vi "Write Stick Deadband.vi"(8 "error in (no error)":errorcluster, 10 "Stick Deadband":dbl, 11 "Joystick in":refnum<class "Joystick.lvclass">) -> (0 "error out":errorcluster, 3 "Joystick out":refnum<class "Joystick.lvclass">)   [LabVIEW 2014, in "Joystick.lvlib" / "Joystick.lvclass"]
uses:
  Joystick.lvclass
  Joystick.lvclass/Joystick.ctl
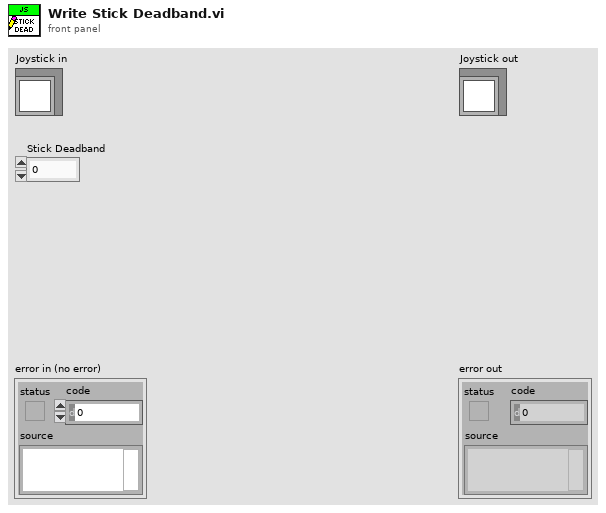
[diagram p1: front panel]
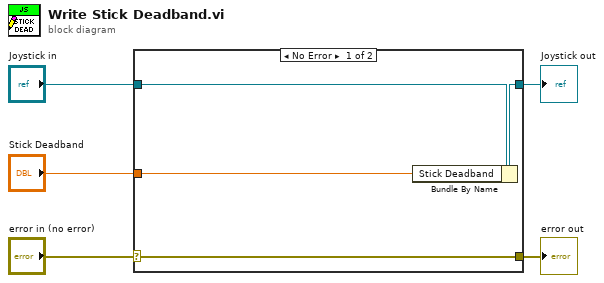
[diagram p0: block diagram]
diagram:
  n1 = case shown="No Error" "error in (no error)" {
    selector: "error in (no error)" -> [w9 w10]
    tunnel: [w9 w10] -> w4
    tunnel: [w7 w11] -> w2
    tunnel: "Joystick in" -> [w8 w11]
    tunnel: "Stick Deadband" -> [w6 _]
    frame No Error {
      n2 = Bundle By Name(cluster=w8, "Stick Deadband"=w6) -> (w7:refnum<class "Joystick.lvclass">)
    }
    frame Error {
    }
  }
  "error out" <- w4
  "Joystick out" <- w2
